vi "Untitled 2.vi"() -> ()   [LabVIEW 2025, in "Data Logger v2.lvlib"]
uses:
  Data Logger v2.lvlib
  TDMS Open Parameters--cluster.ctl
  Write TDMS 2D Array Parameters--cluster.ctl
panel:
  in  "TDMS Write 2D Array Parameters":T1
  out "error out":errorcluster
  in  "TDMS Open Parameters":T2
  in  "error in (no error)":errorcluster
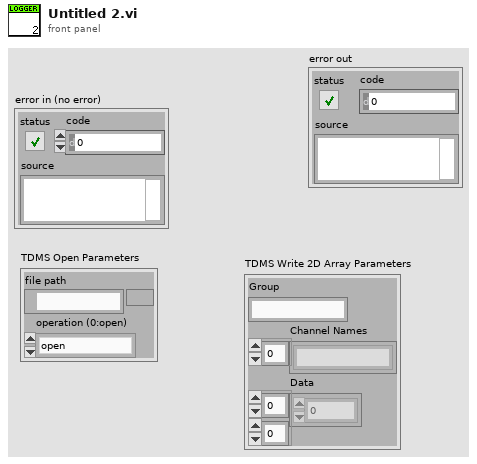
[diagram p1: front panel]
types:
  T1 = typedef "Data Logger v2.lvlib/Write TDMS 2D Array Parameters--cluster.ctl" = cluster{"Group":string, "Channel Names":string[], "Data":dbl[][]}
  T2 = typedef "Data Logger v2.lvlib/TDMS Open Parameters--cluster.ctl" = cluster{"file path":path, "operation (0:open)":enum16{"open", "open or create", "create or replace", "create", "open (read-only)"}}
  T3 = enum16{"open", "open or create", "create or replace", "create", "open (read-only)"}
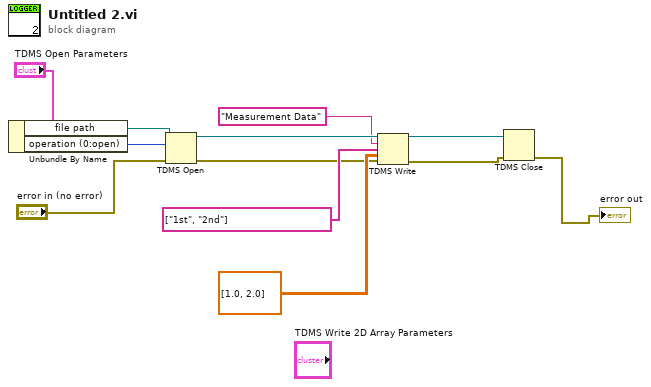
[diagram p0: block diagram]
diagram:
  n1 = Unbundle By Name("TDMS Open Parameters") -> ("file path"=w10:path, "operation (0:open)"=w9:T3)
  n2 = TDMS Open(8:"error in (no error)", 10:w9, 11:w10) -> (0:w2:errorcluster, 3:w8:refnum<k34>)  [unwired: 4 in]
  n3 = TDMS Write(0:w8, 5:"Measurement Data", 7:string[] ["1st", "2nd"], 9:dbl[][] [[1.0], [2.0]], 11:w2) -> (4:w4:refnum<k34>, 15:w3:errorcluster)  [unwired: 1 in, 2 out]
  n4 = TDMS Close(8:w3, 11:w4) -> (0:→"error out":errorcluster)  [unwired: 1 out]
